vi "Bake.vi"(8 "error in (no error)":errorcluster, 11 "Oven in":refnum<class "Oven.lvclass">) -> (0 "error out":errorcluster, 3 "Oven out":refnum<class "Oven.lvclass">)   [LabVIEW 2011, in "Oven.lvclass"]
uses:
  Oven.lvclass
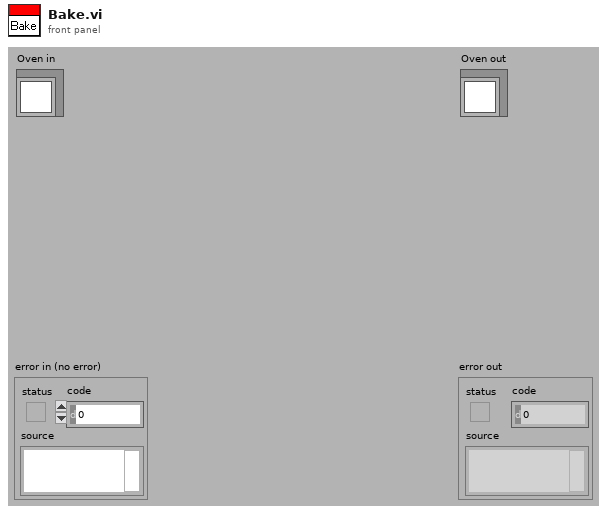
[diagram p1: front panel]
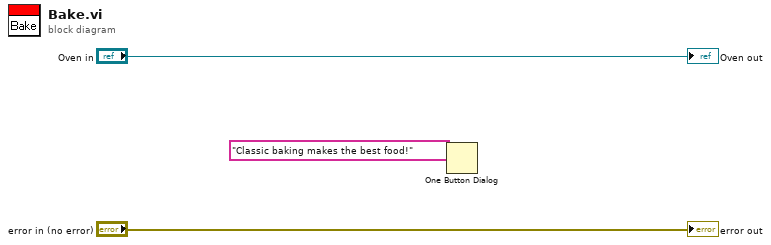
[diagram p0: block diagram]
diagram:
  n1 = One Button Dialog(message="Classic baking makes the best food!") -> ()  [unwired: 1 in, 1 out]
  "error out" <- "error in (no error)"
  "Oven out" <- "Oven in"
